vi "Read_uTTA_CalibrationFile.vi"(8 "error in (no error)":errorcluster, 11 "selected path":path) -> (0 "error out":errorcluster, 1 "PGA":cluster{"Offset":dbl[], "Gain":dbl[]}, 2 "ADC":cluster{"Offset":dbl[], "Gain":dbl[]}, 3 "Channels":T1(array[cluster]))   [LabVIEW 2021]
uses:
  <vilib>/Utility/config.llb/Read Key (Double).vi
  <vilib>/Utility/config.llb/NI_LVConfig.lvlib
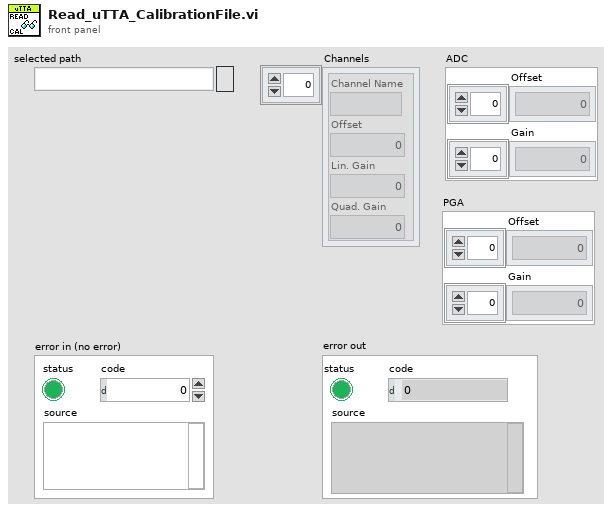
[diagram p1: front panel]
types:
  T1 = cluster{"Channel Name":string, "Offset":dbl, "Lin. Gain":dbl, "Quad. Gain":dbl}[]
  T2 = typedef "NI_LVConfig.lvlib/Config Data RefNum.ctl" = refnum<k1>
  T3 = cluster{"Channel Name":string, "Offset":dbl, "Lin. Gain":dbl, "Quad. Gain":dbl}
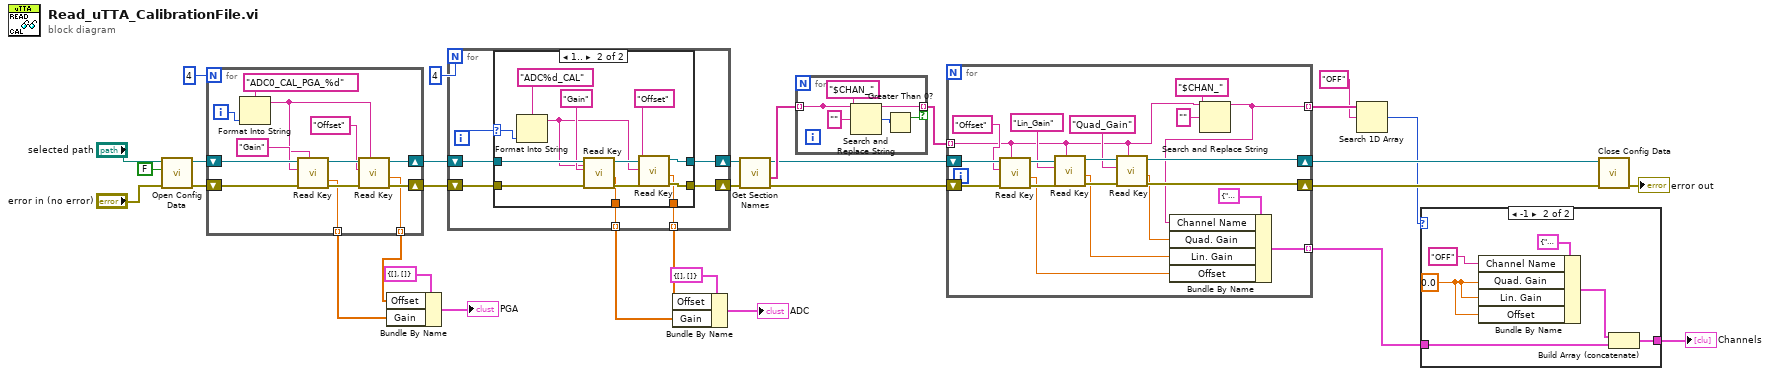
[diagram p0: block diagram]
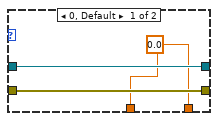
[diagram p3: hidden frame]
diagram:
  n1 = call <vilib>:"Open Config Data.vi"("error in (no error)"="error in (no error)", "create file if necessary (T)"=FALSE, "configuration file path"="selected path") -> ("error out"=w14:errorcluster, "refnum"=w13:T2)  [unwired: 6 in, 1 out]
  n2 = for {
    N: 4 -> [_]
    shift-right: [w35] -> w8
    shift-left: w13 -> [w42]
    shift-right: [w34] -> w7
    shift-left: w14 -> [w41]
    tunnel: [w33] -> w19 mode=indexing
    tunnel: [w32] -> w20 mode=indexing
    i -> [w43]
    n3 = Format Into String(format string="ADC0_CAL_PGA_%d", w43) -> (resulting string=w37:string)  [unwired: 2 in, 1 out]
    n4 = call-poly <vilib>:"Read Key.vi"("section"=w37, "error in (no error)"=w41, "key"="Gain", "refnum"=w42) -> ("error out"=w38:errorcluster, "value"=w32:dbl, "refnum out"=w39:T2)  [unwired: 4 in, 1 out]
    n5 = call-poly <vilib>:"Read Key.vi"("section"=w37, "error in (no error)"=w38, "key"="Offset", "refnum"=w39) -> ("error out"=w34:errorcluster, "value"=w33:dbl, "refnum out"=w35:T2)  [unwired: 4 in, 1 out]
  }
  n6 = Bundle By Name(cluster=cluster{"Offset":dbl[], "Gain":dbl[]} {"Offset"=[], "Gain"=[]} ("input cluster"), "Offset"=w19, "Gain"=w20) -> (→"PGA":cluster{"Offset":dbl[], "Gain":dbl[]})
  n7 = for {
    N: 4 -> [_]
    shift-right: [w49] -> w24
    shift-left: w8 -> [w51]
    shift-right: [w48] -> w25
    shift-left: w7 -> [w50]
    tunnel: [w46] -> w21 mode=indexing
    tunnel: [w45] -> w22 mode=indexing
    i -> [w47]
    n8 = case shown="1.." w47 {
      selector: w47 -> [_ w57]
      tunnel: w51 -> [w54 w66]
      tunnel: w50 -> [w53 w65]
      tunnel: [w54 w59] -> w49
      tunnel: [w53 w58] -> w48
      tunnel: [w52 w56] -> w46
      tunnel: [w52 w55] -> w45
      frame 0, Default {
        w52 = 0.0 ("value")
      }
      frame 1.. {
        n9 = Format Into String(format string="ADC%d_CAL", w57) -> (resulting string=w61:string)  [unwired: 2 in, 1 out]
        n10 = call-poly <vilib>:"Read Key.vi"("section"=w61, "error in (no error)"=w65, "key"="Gain", "refnum"=w66) -> ("error out"=w63:errorcluster, "value"=w55:dbl, "refnum out"=w62:T2)  [unwired: 4 in, 1 out]
        n11 = call-poly <vilib>:"Read Key.vi"("section"=w61, "error in (no error)"=w63, "key"="Offset", "refnum"=w62) -> ("error out"=w58:errorcluster, "value"=w56:dbl, "refnum out"=w59:T2)  [unwired: 4 in, 1 out]
      }
    }
  }
  n12 = Bundle By Name(cluster=cluster{"Offset":dbl[], "Gain":dbl[]} {"Offset"=[], "Gain"=[]} ("input cluster"), "Offset"=w21, "Gain"=w22) -> (→"ADC":cluster{"Offset":dbl[], "Gain":dbl[]})
  n13 = call <vilib>:"Get Section Names.vi"("error in (no error)"=w25, "refnum"=w24) -> ("error out"=w26:errorcluster, "section names"=w28:string[], "refnum out"=w27:T2)  [unwired: 7 in]
  n14 = for {
    tunnel: w28 -> [w68] mode=indexing
    tunnel: [w68] -> w29 mode=indexing if=w69
    n15 = Search and Replace String(input string=w68, search string="$CHAN_" ("string"), replace string="" ("replace string (\"\")")) -> (number of replacements=w70:i32)  [unwired: 5 in, 3 out]
    n16 = Greater Than 0?(x=w70) -> (x > 0?=w69:bool)
  }
  n17 = for {
    shift-right: [w83] -> w15
    shift-left: w27 -> [w92]
    shift-right: [w82] -> w16
    shift-left: w26 -> [w91]
    tunnel: w29 -> [w74] mode=indexing
    tunnel: [w77] -> w5 mode=indexing
    tunnel: [w73] -> w4 mode=indexing
    n18 = call-poly <vilib>:"Read Key.vi"("section"=w74, "error in (no error)"=w91, "key"="Offset", "refnum"=w92) -> ("error out"=w89:errorcluster, "value"=w78:dbl, "refnum out"=w88:T2)  [unwired: 4 in, 1 out]
    n19 = call-poly <vilib>:"Read Key.vi"("section"=w74, "error in (no error)"=w89, "key"="Lin_Gain", "refnum"=w88) -> ("error out"=w85:errorcluster, "value"=w79:dbl, "refnum out"=w86:T2)  [unwired: 4 in, 1 out]
    n20 = call-poly <vilib>:"Read Key.vi"("section"=w74, "error in (no error)"=w85, "key"="Quad_Gain", "refnum"=w86) -> ("error out"=w82:errorcluster, "value"=w80:dbl, "refnum out"=w83:T2)  [unwired: 4 in, 1 out]
    n21 = Search and Replace String(input string=w74, search string="$CHAN_" ("string"), replace string="" ("replace string (\"\")")) -> (result string=w73:string)  [unwired: 5 in, 3 out]
    n22 = Bundle By Name(cluster=T3 {"Channel Name"="", "Offset"=0.0, "Lin. Gain"=0.0, "Quad. Gain"=0.0} ("input cluster"), "Channel Name"=w73, "Quad. Gain"=w80, "Lin. Gain"=w79, "Offset"=w78) -> (w77:T3)
  }
  n23 = Search 1D Array(1D array=w4, element="OFF") -> (index of element=w2:i32)  [unwired: 1 in]
  n24 = case shown="-1" w2 {
    tunnel: w5 -> [w93 w99]
    tunnel: [w93 w98] -> w1
    frame 0, Default {
    }
    frame -1 {
      w95 = 0.0 ("Quad. Gain")
      n25 = Bundle By Name(cluster=T3 {"Channel Name"="", "Offset"=0.0, "Lin. Gain"=0.0, "Quad. Gain"=0.0} ("input cluster"), "Channel Name"="OFF", "Quad. Gain"=w95, "Lin. Gain"=w95, "Offset"=w95) -> (w94:T3)
      n26 = Build Array (concatenate)(w94, w99) -> (w98:T1)
    }
  }
  "Channels" <- w1
  n27 = call <vilib>:"Close Config Data.vi"("error in (no error)"=w16, "refnum"=w15) -> ("error out"=→"error out":errorcluster)  [unwired: 8 in, 1 out]
